vi "JSONtext Multi-step Filter.vi"() -> ()   [LabVIEW 2017] (continued)
laborum. Quis sint fugiat deserunt incididunt enim sit magna occaecat mollit.\\r\\n\",\n    \"registered\": \"2014-01-11T05:01:09 -00:00\",\n    \"latitude\": -55.686363,\n    \"longitude\": -121.895445,\n    \"tags\": [\n      \"nostrud\",\n      \"adipisicing\",\n      \"proident\",\n      \"reprehenderit\",\n      \"minim\",\n      \"incididunt\",\n      \"do\"\n    ],\n    \"friends\": [\n      {\n        \"id\": 0,\n        \"name\": \"Bowman Haynes\"\n      },\n      {\n        \"id\": 1,\n        \"name\": \"Rosalind Dejesus\"\n      },\n      {\n        \"id\": 2,\n        \"name\": \"Mayra Finch\"\n      }\n    ],\n    \"greeting\": \"Hello, Agnes Frye! You have 4 unread messages.\",\n    \"favoriteFruit\": \"apple\"\n  },\n  {\n    \"_id\": \"59b53bcb9737cc098f392507\",\n    \"index\": 79,\n    \"guid\": \"14e019ee-c0ef-4d9f-a34b-1e266fe4f201\",\n    \"isActive\": true,\n    \"balance\": \"$2,153.21\",\n    \"picture\": \"http://placehold.it/32x32\",\n    \"age\": 36,\n    \"eyeColor\": \"blue\",\n    \"name\": \"Edwards Dennis\",\n    \"gender\": \"male\",\n    \"company\": \"ARCTIQ\",\n    \"email\": \"edwardsdennis@arctiq.com\",\n    \"phone\": \"+1 (883) 475-3655\",\n    \"address\": \"269 Melba Court, Soudan, Oregon, 9327\",\n    \"about\": \"Fugiat exercitation sit est excepteur enim culpa. Adipisicing fugiat labore adipisicing fugiat commodo minim. Dolor amet nisi ea deserunt nisi consequat. Duis aliqua in qui veniam exercitation officia labore amet fugiat. Dolore deserunt ullamco quis esse enim incididunt cupidatat. Dolore in laborum dolor id in mollit esse ut sit laborum deserunt duis consequat. Aliqua consectetur nulla esse ad laborum est amet veniam incididunt est anim cillum ad reprehenderit.\\r\\n\",\n    \"registered\": \"2014-11-20T11:02:11 -00:00\",\n    \"latitude\": 4.916048,\n    \"longitude\": 67.818849,\n    \"tags\": [\n      \"ipsum\",\n      \"ea\",\n      \"nisi\",\n      \"fugiat\",\n      \"qui\",\n      \"occaecat\",\n      \"duis\"\n    ],\n    \"friends\": [\n      {\n        \"id\": 0,\n        \"name\": \"Pearson Obrien\"\n      },\n      {\n        \"id\": 1,\n        \"name\": \"Jaime Castillo\"\n      },\n      {\n        \"id\": 2,\n        \"name\": \"Fowler Branch\"\n      }\n    ],\n    \"greeting\": \"Hello, Edwards Dennis! You have 3 unread messages.\",\n    \"favoriteFruit\": \"apple\"\n  },\n  {\n    \"_id\": \"59b53bcbc88425d302bb5dc9\",\n    \"index\": 80,\n    \"guid\": \"8d66411d-3632-46fa-adba-de988295c355\",\n    \"isActive\": true,\n    \"balance\": \"$1,048.45\",\n    \"picture\": \"http://placehold.it/32x32\",\n    \"age\": 20,\n    \"eyeColor\": \"brown\",\n    \"name\": \"Tonya Harrell\",\n    \"gender\": \"female\",\n    \"company\": \"MIRACLIS\",\n    \"email\": \"tonyaharrell@miraclis.com\",\n    \"phone\": \"+1 (955) 521-2821\",\n    \"address\": \"458 Hart Street, Otranto, Florida, 9320\",\n    \"about\": \"Sit laboris tempor do reprehenderit. Reprehenderit exercitation consectetur aliquip nisi nisi occaecat magna magna pariatur. Reprehenderit eiusmod cillum irure aliqua laboris dolore occaecat anim commodo ad dolore. Laborum fugiat minim pariatur sunt enim qui cupidatat labore ex esse cupidatat id aliquip.\\r\\n\",\n    \"registered\": \"2016-08-02T02:36:17 -01:00\",\n    \"latitude\": 60.952856,\n    \"longitude\": 45.278246,\n    \"tags\": [\n      \"minim\",\n      \"nulla\",\n      \"laboris\",\n      \"exercitation\",\n      \"duis\",\n      \"eiusmod\",\n      \"amet\"\n    ],\n    \"friends\": [\n      {\n        \"id\": 0,\n        \"name\": \"Clara Harding\"\n      },\n      {\n        \"id\": 1,\n        \"name\": \"Corine Lindsey\"\n      },\n      {\n        \"id\": 2,\n        \"name\": \"Mcfarland Martinez\"\n      }\n    ],\n    \"greeting\": \"Hello, Tonya Harrell! You have 2 unread messages.\",\n    \"favoriteFruit\": \"strawberry\"\n  },\n  {\n    \"_id\": \"59b53bcb6dc7404c96b23788\",\n    \"index\": 81,\n    \"guid\": \"d16339bd-0d5a-4fda-9a80-3523f38c2607\",\n    \"isActive\": false,\n    \"balance\": \"$3,172.05\",\n    \"picture\": \"http://placehold.it/32x32\",\n    \"age\": 26,\n    \"eyeColor\": \"blue\",\n    \"name\": \"Robertson Malone\",\n    \"gender\": \"male\",\n    \"company\": \"UNIA\",\n    \"email\": \"robertsonmalone@unia.com\",\n    \"phone\": \"+1 (962) 481-2396\",\n    \"address\": \"590 Newel Street, Joppa, Minnesota, 5936\",\n    \"about\": \"Do duis laboris elit dolor amet exercitation. Irure aliqua veniam consectetur culpa enim in officia voluptate ad. Adipisicing sint do et commodo. Culpa in adipisicing voluptate aliqua Lorem exercitation sunt ullamco pariatur voluptate mollit aliquip. Laboris quis labore minim officia. Dolor Lorem tempor aute minim commodo duis incididunt laboris enim sit sint mollit.\\r\\n\",\n    \"registered\": \"2016-07-26T05:07:36 -01:00\",\n    \"latitude\": 74.88141,\n    \"longitude\": -149.072395,\n    \"tags\": [\n      \"sit\",\n      \"commodo\",\n      \"Lorem\",\n      \"ex\",\n      \"fugiat\",\n      \"fugiat\",\n      \"dolor\"\n    ],\n    \"friends\": [\n      {\n        \"id\": 0,\n        \"name\": \"Winifred Tate\"\n      },\n      {\n        \"id\": 1,\n        \"name\": \"Curtis Reid\"\n      },\n      {\n        \"id\": 2,\n        \"name\": \"Chase Keith\"\n      }\n    ],\n    \"greeting\": \"Hello, Robertson Malone! You have 7 unread messages.\",\n    \"favoriteFruit\": \"apple\"\n  },\n  {\n    \"_id\": \"59b53bcb51c65aa434aa3d1f\",\n    \"index\": 82,\n    \"guid\": \"2774080d-3b85-4a4f-97f3-157e9148c011\",\n    \"isActive\": true,\n    \"balance\": \"$3,693.94\",\n    \"picture\": \"http://placehold.it/32x32\",\n    \"age\": 21,\n    \"eyeColor\": \"blue\",\n    \"name\": \"Mercedes Leonard\",\n    \"gender\": \"female\",\n    \"company\": \"MIRACULA\",\n    \"email\": \"mercedesleonard@miracula.com\",\n    \"phone\": \"+1 (847) 435-3340\",\n    \"address\": \"900 Grafton Street, Mulberry, Hawaii, 4401\",\n    \"about\": \"Consectetur laborum eu occaecat occaecat id minim. Duis do veniam adipisicing voluptate consectetur labore quis elit. Cillum dolore ex fugiat deserunt sint ea magna cillum reprehenderit amet consectetur proident. Culpa ut cillum nulla sit voluptate voluptate veniam qui. Ut anim minim pariatur velit dolor cupidatat ut. Irure Lorem fugiat incididunt ad cillum sit nisi sunt sint dolor elit. Elit non minim laborum ex dolor commodo labore quis irure officia duis labore.\\r\\n\",\n    \"registered\": \"2015-09-07T03:13:08 -01:00\",\n    \"latitude\": -37.746734,\n    \"longitude\": 158.145458,\n    \"tags\": [\n      \"ipsum\",\n      \"dolor\",\n      \"occaecat\",\n      \"aute\",\n      \"dolor\",\n      \"ex\",\n      \"id\"\n    ],\n    \"friends\": [\n      {\n        \"id\": 0,\n        \"name\": \"Jerri Miller\"\n      },\n      {\n        \"id\": 1,\n        \"name\": \"Huff Pitts\"\n      },\n      {\n        \"id\": 2,\n        \"name\": \"Kristine Pittman\"\n      }\n    ],\n    \"greeting\": \"Hello, Mercedes Leonard! You have 7 unread messages.\",\n    \"favoriteFruit\": \"apple\"\n  },\n  {\n    \"_id\": \"59b53bcbb5cb7bde1ba115a7\",\n    \"index\": 83,\n    \"guid\": \"5fa9bb18-fd83-47f9-8f54-1c8eab99fa1f\",\n    \"isActive\": false,\n    \"balance\": \"$2,449.67\",\n    \"picture\": \"http://placehold.it/32x32\",\n    \"age\": 27,\n    \"eyeColor\": \"brown\",\n    \"name\": \"Rebekah Cardenas\",\n    \"gender\": \"female\",\n    \"company\": \"MEDCOM\",\n    \"email\": \"rebekahcardenas@medcom.com\",\n    \"phone\": \"+1 (930) 526-2666\",\n    \"address\": \"585 Conduit Boulevard, Edenburg, Pennsylvania, 5520\",\n    \"about\": \"Sint magna ad consequat cupidatat ut quis duis ut deserunt duis sit consequat. Nisi ea ad ex occaecat adipisicing voluptate quis aliquip nostrud amet quis. Veniam consectetur amet magna adipisicing commodo ea esse elit occaecat labore pariatur. Adipisicing laboris Lorem sit incididunt pariatur eu. Do ipsum laborum excepteur cillum in.\\r\\n\",\n    \"registered\": \"2015-04-23T12:08:15 -01:00\",\n    \"latitude\": -70.810485,\n    \"longitude\": -5.673714,\n    \"tags\": [\n      \"eu\",\n      \"elit\",\n      \"do\",\n      \"laboris\",\n      \"eu\",\n      \"pariatur\",\n      \"sunt\"\n    ],\n    \"friends\": [\n      {\n        \"id\": 0,\n        \"name\": \"Selma Hughes\"\n      },\n      {\n        \"id\": 1,\n        \"name\": \"Laverne Ware\"\n      },\n      {\n        \"id\": 2,\n        \"name\": \"Cortez Reilly\"\n      }\n    ],\n    \"greeting\": \"Hello, Rebekah Cardenas! You have 5 unread messages.\",\n    \"favoriteFruit\": \"strawberry\"\n  },\n  {\n    \"_id\": \"59b53bcbf398f609774512fb\",\n    \"index\": 84,\n    \"guid\": \"9798106c-d85b-4df5-a840-9220e34cb34d\",\n    \"isActive\": true,\n    \"balance\": \"$3,845.69\",\n    \"picture\": \"http://placehold.it/32x32\",\n    \"age\": 28,\n    \"eyeColor\": \"brown\",\n    \"name\": \"Rena Norman\",\n    \"gender\": \"female\",\n    \"company\": \"AQUOAVO\",\n    \"email\": \"renanorman@aquoavo.com\",\n    \"phone\": \"+1 (983) 520-2908\",\n    \"address\": \"635 Cedar Street, Richford, Virginia, 7412\",\n    \"about\": \"Id incididunt in veniam officia nisi veniam dolore laboris duis. Eu dolore labore excepteur tempor exercitation pariatur est commodo elit ullamco quis voluptate. Culpa magna anim ad nisi cupidatat proident dolor sit esse aute reprehenderit deserunt id non. Aliquip consequat nulla aliqua mollit dolore nostrud officia amet pariatur commodo proident. Dolore occaecat ex cupidatat ea exercitation velit amet. Laborum officia non anim ea eiusmod tempor consequat laboris est enim culpa irure enim. Sit dolor dolore dolore nisi magna deserunt sint culpa est excepteur aute.\\r\\n\",\n    \"registered\": \"2015-12-14T03:36:58 -00:00\",\n    \"latitude\": -35.296091,\n    \"longitude\": 130.813918,\n    \"tags\": [\n      \"laboris\",\n      \"nisi\",\n      \"ipsum\",\n      \"qui\",\n      \"reprehenderit\",\n      \"ipsum\",\n      \"incididunt\"\n    ],\n    \"friends\": [\n      {\n        \"id\": 0,\n        \"name\": \"Fry Pace\"\n      },\n      {\n        \"id\": 1,\n        \"name\": \"Levy Norton\"\n      },\n      {\n        \"id\": 2,\n        \"name\": \"Lupe Snider\"\n      }\n    ],\n    \"greeting\": \"Hello, Rena Norman! You have 3 unread messages.\",\n    \"favoriteFruit\": \"banana\"\n  },\n  {\n    \"_id\": \"59b53bcb388b74959570b328\",\n    \"index\": 85,\n    \"guid\": \"ef150b45-285d-447c-8120-8e1ae6b7ddb0\",\n    \"isActive\": false,\n    \"balance\": \"$3,528.91\",\n    \"picture\": \"http://placehold.it/32x32\",\n    \"age\": 33,\n    \"eyeColor\": \"green\",\n    \"name\": \"Russell Hunter\",\n    \"gender\": \"male\",\n    \"company\": \"KONNECT\",\n    \"email\": \"russellhunter@konnect.com\",\n    \"phone\": \"+1 (923) 579-2669\",\n    \"address\": \"991 Agate Court, Westwood, Kansas, 7904\",\n    \"about\": \"Mollit officia duis anim laborum et sunt dolor commodo est fugiat. Cillum ipsum minim irure ea pariatur officia non deserunt aliqua sit Lorem veniam. Cillum amet deserunt occaecat eiusmod magna esse mollit. Eiusmod fugiat et cillum minim ullamco velit sint enim qui exercitation. Magna nostrud deserunt adipisicing nisi ullamco quis culpa aliquip voluptate do.\\r\\n\",\n    \"registered\": \"2014-01-24T12:47:30 -00:00\",\n    \"latitude\": -4.402596,\n    \"longitude\": -44.068437,\n    \"tags\": [\n      \"duis\",\n      \"aliqua\",\n      \"aliquip\",\n      \"ullamco\",\n      \"nulla\",\n      \"anim\",\n      \"eiusmod\"\n    ],\n    \"friends\": [\n      {\n        \"id\": 0,\n        \"name\": \"Jolene Bonner\"\n      },\n      {\n        \"id\": 1,\n        \"name\": \"Head Calhoun\"\n      },\n      {\n        \"id\": 2,\n        \"name\": \"Kate Reyes\"\n      }\n    ],\n    \"greeting\": \"Hello, Russell Hunter! You have 6 unread messages.\",\n    \"favoriteFruit\": \"strawberry\"\n  },\n  {\n    \"_id\": \"59b53bcb2db0467411e874a7\",\n    \"index\": 86,\n    \"guid\": \"c8749167-fdd7-4919-911e-bf0b7c47fa22\",\n    \"isActive\": true,\n    \"balance\": \"$3,021.98\",\n    \"picture\": \"http://placehold.it/32x32\",\n    \"age\": 30,\n    \"eyeColor\": \"green\",\n    \"name\": \"Singleton May\",\n    \"gender\": \"male\",\n    \"company\": \"OBONES\",\n    \"email\": \"singletonmay@obones.com\",\n    \"phone\": \"+1 (809) 470-2340\",\n    \"address\": \"513 Stuyvesant Avenue, Fairlee, Puerto Rico, 6772\",\n    \"about\": \"Ea irure Lorem nulla duis do do et nostrud exercitation. Voluptate exercitation aute consequat eu est. Et cillum labore consectetur amet. Ea pariatur magna et excepteur anim sit pariatur occaecat velit sunt veniam anim.\\r\\n\",\n    \"registered\": \"2016-04-15T10:43:19 -01:00\",\n    \"latitude\": -67.961908,\n    \"longitude\": -28.926166,\n    \"tags\": [\n      \"consequat\",\n      \"pariatur\",\n      \"tempor\",\n      \"et\",\n      \"excepteur\",\n      \"incididunt\",\n      \"tempor\"\n    ],\n    \"friends\": [\n      {\n        \"id\": 0,\n        \"name\": \"Mendoza Estes\"\n      },\n      {\n        \"id\": 1,\n        \"name\": \"Bean Bolton\"\n      },\n      {\n        \"id\": 2,\n        \"name\": \"Holder Villarreal\"\n      }\n    ],\n    \"greeting\": \"Hello, Singleton May! You have 3 unread messages.\",\n    \"favoriteFruit\": \"apple\"\n  },\n  {\n    \"_id\": \"59b53bcbaefe5ada14509d19\",\n    \"index\": 87,\n    \"guid\": \"ead04019-6a40-4420-a798-b8883cd03185\",\n    \"isActive\": true,\n    \"balance\": \"$1,396.19\",\n    \"picture\": \"http://placehold.it/32x32\",\n    \"age\": 39,\n    \"eyeColor\": \"blue\",\n    \"name\": \"Jewell Bradshaw\",\n    \"gender\": \"female\",\n    \"company\": \"JUMPSTACK\",\n    \"email\": \"jewellbradshaw@jumpstack.com\",\n    \"phone\": \"+1 (968) 458-2531\",\n    \"address\": \"782 Winthrop Street, Dotsero, South Carolina, 5062\",\n    \"about\": \"Amet deserunt pariatur in elit exercitation labore. Quis dolore Lorem pariatur irure tempor amet culpa duis enim deserunt exercitation proident. Nostrud magna qui irure dolore est excepteur magna nulla ipsum anim ullamco. Velit occaecat sunt exercitation minim consequat. Eu sunt cillum non amet pariatur mollit sunt amet ad non irure.\\r\\n\",\n    \"registered\": \"2014-09-14T04:22:20 -01:00\",\n    \"latitude\": 29.814291,\n    \"longitude\": 61.37831,\n    \"tags\": [\n      \"sint\",\n      \"elit\",\n      \"ad\",\n      \"ad\",\n      \"cupidatat\",\n      \"cillum\",\n      \"sit\"\n    ],\n    \"friends\": [\n      {\n        \"id\": 0,\n        \"name\": \"Rosales Richmond\"\n      },\n      {\n        \"id\": 1,\n        \"name\": \"Sara Duffy\"\n      },\n      {\n        \"id\": 2,\n        \"name\": \"Freida Pollard\"\n      }\n    ],\n    \"greeting\": \"Hello, Jewell Bradshaw! You have 10 unread messages.\",\n    \"favoriteFruit\": \"strawberry\"\n  },\n  {\n    \"_id\": \"59b53bcb431347b2e14132f2\",\n    \"index\": 88,\n    \"guid\": \"caf8be88-33b4-4c13-8fba-e0e573a30583\",\n    \"isActive\": true,\n    \"balance\": \"$1,502.06\",\n    \"picture\": \"http://placehold.it/32x32\",\n    \"age\": 40,\n    \"eyeColor\": \"blue\",\n    \"name\": \"Langley Bauer\",\n    \"gender\": \"male\",\n    \"company\": \"PORTICA\",\n    \"email\": \"langleybauer@portica.com\",\n    \"phone\": \"+1 (980) 600-2629\",\n    \"address\": \"193 George Street, Navarre, Mississippi, 3789\",\n    \"about\": \"Exercitation irure ad magna sunt consequat non. Do amet tempor consequat adipisicing reprehenderit sunt. Do ipsum aliquip dolore amet ullamco. Eu proident reprehenderit consequat velit. Exercitation minim eiusmod quis incididunt magna magna exercitation consectetur irure.\\r\\n\",\n    \"registered\": \"2015-12-09T03:10:32 -00:00\",\n    \"latitude\": 14.711439,\n    \"longitude\": 101.330203,\n    \"tags\": [\n      \"sunt\",\n      \"laboris\",\n      \"nisi\",\n      \"velit\",\n      \"ipsum\",\n      \"fugiat\",\n      \"amet\"\n    ],\n    \"friends\": [\n      {\n        \"id\": 0,\n        \"name\": \"Noble Odom\"\n      },\n      {\n        \"id\": 1,\n        \"name\": \"Mara Everett\"\n      },\n      {\n        \"id\": 2,\n        \"name\": \"Carole Benson\"\n      }\n    ],\n    \"greeting\": \"Hello, Langley Bauer! You have 1 unread messages.\",\n    \"favoriteFruit\": \"apple\"\n  },\n  {\n    \"_id\": \"59b53bcb9cfbbb3d3b86db36\",\n    \"index\": 89,\n    \"guid\": \"585ace61-13af-493d-9fa6-61d9246efb80\",\n    \"isActive\": true,\n    \"balance\": \"$2,788.64\",\n    \"picture\": \"http://placehold.it/32x32\",\n    \"age\": 39,\n    \"eyeColor\": \"green\",\n    \"name\": \"Walker Sandoval\",\n    \"gender\": \"male\",\n    \"company\": \"EXPOSA\",\n    \"email\": \"walkersandoval@exposa.com\",\n    \"phone\": \"+1 (813) 589-3863\",\n    \"address\": \"597 Dunham Place, Albrightsville, Wisconsin, 6040\",\n    \"about\": \"Cillum ipsum velit ea esse cupidatat aliquip deserunt. Velit labore enim et et dolor esse duis voluptate Lorem ea. Esse Lorem excepteur quis cillum mollit anim voluptate fugiat est culpa. Ullamco Lorem fugiat tempor sunt incididunt aliquip occaecat mollit sit aliqua velit. Ex ullamco consequat minim minim do sint commodo anim fugiat do. Cupidatat id nulla in adipisicing magna consequat deserunt cillum. Ad id occaecat mollit id ullamco.\\r\\n\",\n    \"registered\": \"2016-04-14T12:25:38 -01:00\",\n    \"latitude\": -16.535757,\n    \"longitude\": -28.076556,\n    \"tags\": [\n      \"consectetur\",\n      \"commodo\",\n      \"magna\",\n      \"duis\",\n      \"cillum\",\n      \"id\",\n      \"mollit\"\n    ],\n    \"friends\": [\n      {\n        \"id\": 0,\n        \"name\": \"Tamra Watson\"\n      },\n      {\n        \"id\": 1,\n        \"name\": \"Deidre Gamble\"\n      },\n      {\n        \"id\": 2,\n        \"name\": \"Graham Harris\"\n      }\n    ],\n    \"greeting\": \"Hello, Walker Sandoval! You have 6 unread messages.\",\n    \"favoriteFruit\": \"banana\"\n  },\n  {\n    \"_id\": \"59b53bcb4f8125393e1be565\",\n    \"index\": 90,\n    \"guid\": \"50b5a169-63ec-430b-bd65-956e383c7b25\",\n    \"isActive\": true,\n    \"balance\": \"$2,863.84\",\n    \"picture\": \"http://placehold.it/32x32\",\n    \"age\": 33,\n    \"eyeColor\": \"brown\",\n    \"name\": \"Carlene Humphrey\",\n    \"gender\": \"female\",\n    \"company\": \"WEBIOTIC\",\n    \"email\": \"carlenehumphrey@webiotic.com\",\n    \"phone\": \"+1 (957) 535-2883\",\n    \"address\": \"367 Kensington Street, Carrizo, Indiana, 3136\",\n    \"about\": \"Voluptate pariatur ex pariatur duis non quis ex cillum. Labore occaecat tempor in enim proident aliquip. Consequat ex veniam ullamco aute aute cupidatat dolor dolore ad velit incididunt.\\r\\n\",\n    \"registered\": \"2015-09-17T11:41:14 -01:00\",\n    \"latitude\": -25.860369,\n    \"longitude\": 159.878255,\n    \"tags\": [\n      \"eiusmod\",\n      \"consectetur\",\n      \"consectetur\",\n      \"id\",\n      \"id\",\n      \"eiusmod\",\n      \"ad\"\n    ],\n    \"friends\": [\n      {\n        \"id\": 0,\n        \"name\": \"Baird Reed\"\n      },\n      {\n        \"id\": 1,\n        \"name\": \"Dollie Stephens\"\n      },\n      {\n        \"id\": 2,\n        \"name\": \"Greta Buckley\"\n      }\n    ],\n    \"greeting\": \"Hello, Carlene Humphrey! You have 6 unread messages.\",\n    \"favoriteFruit\": \"banana\"\n  },\n  {\n    \"_id\": \"59b53bcb68c2646e78378cd5\",\n    \"index\": 91,\n    \"guid\": \"ea0a37f9-d18f-4eba-8810-ab098ee81cd3\",\n    \"isActive\": true,\n    \"balance\": \"$1,333.07\",\n    \"picture\": \"http://placehold.it/32x32\",\n    \"age\": 22,\n    \"eyeColor\": \"brown\",\n    \"name\": \"Mattie Mckinney\",\n    \"gender\": \"female\",\n    \"company\": \"PATHWAYS\",\n    \"email\": \"mattiemckinney@pathways.com\",\n    \"phone\": \"+1 (985) 530-3103\",\n    \"address\": \"803 Taaffe Place, Brutus, Tennessee, 1065\",\n    \"about\": \"Aute aute ipsum nostrud commodo. Elit laboris magna irure id laboris eu et nisi. Sit ipsum irure deserunt voluptate nisi ut ut. Aute ullamco deserunt ex elit in et qui excepteur aliquip. Dolore id veniam irure irure anim irure ex exercitation id ea.\\r\\n\",\n    \"registered\": \"2014-11-08T08:00:06 -00:00\",\n    \"latitude\": -3.533773,\n    \"longitude\": -136.23028,\n    \"tags\": [\n      \"sit\",\n      \"excepteur\",\n      \"esse\",\n      \"fugiat\",\n      \"proident\",\n      \"id\",\n      \"veniam\"\n    ],\n    \"friends\": [\n      {\n        \"id\": 0,\n        \"name\": \"Latonya Wright\"\n      },\n      {\n        \"id\": 1,\n        \"name\": \"Mable Estrada\"\n      },\n      {\n        \"id\": 2,\n        \"name\": \"Estelle Henson\"\n      }\n    ],\n    \"greeting\": \"Hello, Mattie Mckinney! You have 2 unread messages.\",\n    \"favoriteFruit\": \"strawberry\"\n  },\n  {\n    \"_id\": \"59b53bcb88186672d782d77f\",\n    \"index\": 92,\n    \"guid\": \"63483e35-f63f-47ea-904f-a48dcde71fb1\",\n    \"isActive\": false,\n    \"balance\": \"$3,958.35\",\n    \"picture\": \"http://placehold.it/32x32\",\n    \"age\": 22,\n    \"eyeColor\": \"green\",\n    \"name\": \"Tamara Russo\",\n    \"gender\": \"female\",\n    \"company\": \"EBIDCO\",\n    \"email\": \"tamararusso@ebidco.com\",\n    \"phone\": \"+1 (941) 482-2355\",\n    \"address\": \"184 Dumont Avenue, Chumuckla, Georgia, 7344\",\n    \"about\": \"Tempor cupidatat labore excepteur irure velit sunt aliqua aliquip ea qui. Deserunt mollit cupidatat non amet exercitation eu proident. Occaecat excepteur aliqua exercitation irure dolor. Eiusmod adipisicing incididunt reprehenderit anim proident nulla cupidatat anim. In non consectetur laborum adipisicing nostrud. Eiusmod mollit voluptate aute et ut est voluptate enim laborum occaecat incididunt.\\r\\n\",\n    \"registered\": \"2014-01-11T06:03:38 -00:00\",\n    \"latitude\": 4.570218,\n    \"longitude\": 97.967557,\n    \"tags\": [\n      \"adipisicing\",\n      \"occaecat\",\n      \"tempor\",\n      \"anim\",\n      \"commodo\",\n      \"do\",\n      \"ea\"\n    ],\n    \"friends\": [\n      {\n        \"id\": 0,\n        \"name\": \"Suzette Burch\"\n      },\n      {\n        \"id\": 1,\n        \"name\": \"Velazquez Mayer\"\n      },\n      {\n        \"id\": 2,\n        \"name\": \"Shannon Powell\"\n      }\n    ],\n    \"greeting\": \"Hello, Tamara Russo! You have 9 unread messages.\",\n    \"favoriteFruit\": \"banana\"\n  },\n  {\n    \"_id\": \"59b53bcb9c166135e4f617f9\",\n    \"index\": 93,\n    \"guid\": \"93bacd52-b79c-429e-8685-45799e149002\",\n    \"isActive\": false,\n    \"balance\": \"$2,892.53\",\n    \"picture\": \"http://placehold.it/32x32\",\n    \"age\": 22,\n    \"eyeColor\": \"brown\",\n    \"name\": \"Camacho Talley\",\n    \"gender\": \"male\",\n    \"company\": \"GRAINSPOT\",\n    \"email\": \"camachotalley@grainspot.com\",\n    \"phone\": \"+1 (877) 502-3157\",\n    \"address\": \"977 Roosevelt Court, Gila, New Hampshire, 5370\",\n    \"about\": \"Duis nulla culpa cupidatat amet amet qui. Ut sit dolor laboris quis ullamco. Aute nulla aliqua voluptate fugiat labore ut. Sunt veniam veniam duis commodo pariatur. Commodo occaecat anim ad est aliquip.\\r\\n\",\n    \"registered\": \"2014-09-29T05:59:11 -01:00\",\n    \"latitude\": 65.471967,\n    \"longitude\": -142.24607,\n    \"tags\": [\n      \"id\",\n      \"aute\",\n      \"magna\",\n      \"eiusmod\",\n      \"mollit\",\n      \"ipsum\",\n      \"commodo\"\n    ],\n    \"friends\": [\n      {\n        \"id\": 0,\n        \"name\": \"Hopkins Atkins\"\n      },\n      {\n        \"id\": 1,\n        \"name\": \"Mcclain Santos\"\n      },\n      {\n        \"id\": 2,\n        \"name\": \"Enid Kemp\"\n      }\n    ],\n    \"greeting\": \"Hello, Camacho Talley! You have 5 unread messages.\",\n    \"favoriteFruit\": \"strawberry\"\n  },\n  {\n    \"_id\": \"59b53bcbe2a5bd209ec5b3c8\",\n    \"index\": 94,\n    \"guid\": \"036605db-b6ec-42e9-a1bc-ee2f3b70a5df\",\n    \"isActive\": false,\n    \"balance\": \"$3,938.69\",\n    \"picture\": \"http://placehold.it/32x32\",\n    \"age\": 38,\n    \"eyeColor\": \"green\",\n    \"name\": \"Barbra Morton\",\n    \"gender\": \"female\",\n    \"company\": \"DANJA\",\n    \"email\": \"barbramorton@danja.com\",\n    \"phone\": \"+1 (948) 444-3914\",\n    \"address\": \"970 Rutherford Place, Selma, Louisiana, 3091\",\n    \"about\": \"Proident labore esse non enim consequat laboris quis irure pariatur enim. Aliquip veniam id occaecat laborum consectetur proident ea cillum amet consequat in id. Esse fugiat veniam ullamco culpa exercitation. Pariatur deserunt consectetur qui consectetur aliquip ea irure eiusmod. Ipsum sint ad ex id. Veniam laborum quis cillum qui quis exercitation qui aliquip mollit eiusmod.\\r\\n\",\n    \"registered\": \"2017-08-11T12:43:09 -01:00\",\n    \"latitude\": 36.516788,\n    \"longitude\": 150.180024,\n    \"tags\": [\n      \"tempor\",\n      \"id\",\n      \"aliquip\",\n      \"sit\",\n      \"dolore\",\n      \"qui\",\n      \"nulla\"\n    ],\n    \"friends\": [\n      {\n        \"id\": 0,\n        \"name\": \"Benton Boyle\"\n      },\n      {\n        \"id\": 1,\n        \"name\": \"Bates Mejia\"\n      },\n      {\n        \"id\": 2,\n        \"name\": \"Montoya Weber\"\n      }\n    ],\n    \"greeting\": \"Hello, Barbra Morton! You have 3 unread messages.\",\n    \"favoriteFruit\": \"strawberry\"\n  },\n  {\n    \"_id\": \"59b53bcb7e036dc098f119d8\",\n    \"index\": 95,\n    \"guid\": \"acd5167b-c778-494e-9b08-c3867c5930d5\",\n    \"isActive\": true,\n    \"balance\": \"$3,887.96\",\n    \"picture\": \"http://placehold.it/32x32\",\n    \"age\": 28,\n    \"eyeColor\": \"blue\",\n    \"name\": \"Andrea Barton\",\n    \"gender\": \"female\",\n    \"company\": \"TRIPSCH\",\n    \"email\": \"andreabarton@tripsch.com\",\n    \"phone\": \"+1 (839) 508-3740\",\n    \"address\": \"531 Elm Place, Choctaw, Oklahoma, 4348\",\n    \"about\": \"Aute ullamco laborum esse quis voluptate enim amet consectetur non incididunt nostrud anim sit ea. Quis eiusmod reprehenderit tempor ea aliquip. Magna laboris pariatur id aliqua nostrud labore incididunt ut.\\r\\n\",\n    \"registered\": \"2017-01-18T09:09:30 -00:00\",\n    \"latitude\": 87.073078,\n    \"longitude\": -153.089878,\n    \"tags\": [\n      \"minim\",\n      \"deserunt\",\n      \"proident\",\n      \"dolore\",\n      \"sunt\",\n      \"excepteur\",\n      \"ea\"\n    ],\n    \"friends\": [\n      {\n        \"id\": 0,\n        \"name\": \"Samantha Carrillo\"\n      },\n      {\n        \"id\": 1,\n        \"name\": \"Burke Mckenzie\"\n      },\n      {\n        \"id\": 2,\n        \"name\": \"Alford Love\"\n      }\n    ],\n    \"greeting\": \"Hello, Andrea Barton! You have 6 unread messages.\",\n    \"favoriteFruit\": \"strawberry\"\n  },\n  {\n    \"_id\": \"59b53bcbe68489b710be92d8\",\n    \"index\": 96,\n    \"guid\": \"fcdbceb5-35bc-464d-9cda-0730a96ae61d\",\n    \"isActive\": false,\n    \"balance\": \"$3,067.07\",\n    \"picture\": \"http://placehold.it/32x32\",\n    \"age\": 29,\n    \"eyeColor\": \"blue\",\n    \"name\": \"Edna Simpson\",\n    \"gender\": \"female\",\n    \"company\": \"TYPHONICA\",\n    \"email\": \"ednasimpson@typhonica.com\",\n    \"phone\": \"+1 (887) 582-2829\",\n    \"address\": \"169 Dictum Court, Callaghan, Alaska, 6930\",\n    \"about\": \"Elit veniam ea culpa do nulla consequat culpa ad sunt enim. Laborum aliqua voluptate incididunt magna aliqua consectetur officia consequat anim fugiat aliquip proident cillum. Sunt proident occaecat dolore aute tempor labore minim consectetur. Esse mollit velit id aute minim eiusmod labore cillum. Adipisicing aliquip minim cupidatat nulla aliquip eiusmod quis ut nulla occaecat nulla cupidatat. Tempor laboris consectetur reprehenderit mollit eu cillum pariatur laboris commodo enim Lorem officia.\\r\\n\",\n    \"registered\": \"2016-05-10T05:37:46 -01:00\",\n    \"latitude\": -30.023422,\n    \"longitude\": 0.886087,\n    \"tags\": [\n      \"in\",\n      \"id\",\n      \"officia\",\n      \"anim\",\n      \"labore\",\n      \"ad\",\n      \"sunt\"\n    ],\n    \"friends\": [\n      {\n        \"id\": 0,\n        \"name\": \"Lina Brown\"\n      },\n      {\n        \"id\": 1,\n        \"name\": \"Cain Campos\"\n      },\n      {\n        \"id\": 2,\n        \"name\": \"Sparks Jones\"\n      }\n    ],\n    \"greeting\": \"Hello, Edna Simpson! You have 10 unread messages.\",\n    \"favoriteFruit\": \"banana\"\n  },\n  {\n    \"_id\": \"59b53bcbcfbbc8d0511541f4\",\n    \"index\": 97,\n    \"guid\": \"7281cfd2-d40d-48e4-957e-b86b371683a2\",\n    \"isActive\": true,\n    \"balance\": \"$2,179.76\",\n    \"picture\": \"http://placehold.it/32x32\",\n    \"age\": 35,\n    \"eyeColor\": \"brown\",\n    \"name\": \"Charlene Woods\",\n    \"gender\": \"female\",\n    \"company\": \"JUNIPOOR\",\n    \"email\": \"charlenewoods@junipoor.com\",\n    \"phone\": \"+1 (919) 557-3560\",\n    \"address\": \"161 Tabor Court, Itmann, North Dakota, 9686\",\n    \"about\": \"Mollit velit cillum irure Lorem id consectetur fugiat. Reprehenderit ipsum aliquip tempor dolor. Eu reprehenderit tempor adipisicing anim duis non quis officia excepteur fugiat sunt adipisicing. Consectetur qui aliquip eiusmod laborum do incididunt id ipsum sint est elit ad commodo. Adipisicing veniam eu tempor id et nisi fugiat. Qui duis aute fugiat qui ut id ut deserunt adipisicing aliqua. Fugiat aliqua incididunt Lorem esse ipsum elit magna quis eiusmod pariatur.\\r\\n\",\n    \"registered\": \"2014-09-19T12:55:15 -01:00\",\n    \"latitude\": 23.852484,\n    \"longitude\": 64.974725,\n    \"tags\": [\n      \"deserunt\",\n      \"pariatur\",\n      \"nulla\",\n      \"qui\",\n      \"nulla\",\n      \"proident\",\n      \"aliquip\"\n    ],\n    \"friends\": [\n      {\n        \"id\": 0,\n        \"name\": \"Rachael Cabrera\"\n      },\n      {\n        \"id\": 1,\n        \"name\": \"Best Huber\"\n      },\n      {\n        \"id\": 2,\n        \"name\": \"Luann Abbott\"\n      }\n    ],\n    \"greeting\": \"Hello, Charlene Woods! You have 2 unread messages.\",\n    \"favoriteFruit\": \"banana\"\n  },\n  {\n    \"_id\": \"59b53bcb678a7787e8012db4\",\n    \"index\": 98,\n    \"guid\": \"7519df16-5d86-4a4e-a0b6-19e2f100d49d\",\n    \"isActive\": true,\n    \"balance\": \"$3,153.52\",\n    \"picture\": \"http://placehold.it/32x32\",\n    \"age\": 31,\n    \"eyeColor\": \"blue\",\n    \"name\": \"Pugh Christensen\",\n    \"gender\": \"male\",\n    \"company\": \"PLEXIA\",\n    \"email\": \"pughchristensen@plexia.com\",\n    \"phone\": \"+1 (803) 541-2906\",\n    \"address\": \"514 Wyckoff Avenue, Concho, Washington, 1004\",\n    \"about\": \"Fugiat duis nisi esse duis ut tempor laborum amet. Ut et labore quis pariatur ullamco deserunt esse occaecat est pariatur. Ut cillum pariatur nulla dolor eu consequat nisi nisi occaecat occaecat ad veniam commodo. Cillum anim eu fugiat minim excepteur dolor sit. Dolore aute ipsum qui magna cillum ipsum enim aute ex. Sint veniam deserunt id do velit eu.\\r\\n\",\n    \"registered\": \"2016-10-15T11:07:09 -01:00\",\n    \"latitude\": -71.61758,\n    \"longitude\": -73.196318,\n    \"tags\": [\n      \"pariatur\",\n      \"officia\",\n      \"do\",\n      \"est\",\n      \"aute\",\n      \"ipsum\",\n      \"elit\"\n    ],\n    \"friends\": [\n      {\n        \"id\": 0,\n        \"name\": \"Todd Mccray\"\n      },\n      {\n        \"id\": 1,\n        \"name\": \"Carrillo Johns\"\n      },\n      {\n        \"id\": 2,\n        \"name\": \"Claire Evans\"\n      }\n    ],\n    \"greeting\": \"Hello, Pugh Christensen! You have 6 unread messages.\",\n    \"favoriteFruit\": \"strawberry\"\n  },\n  {\n    \"_id\": \"59b53bcb07c3d92599f358a7\",\n    \"index\": 99,\n    \"guid\": \"00eb41e9-cb16-49c9-84da-e139407a70e3\",\n    \"isActive\": true,\n    \"balance\": \"$3,233.68\",\n    \"picture\": \"http://placehold.it/32x32\",\n    \"age\": 37,\n    \"eyeColor\": \"blue\",\n    \"name\": \"Knapp Mccullough\",\n    \"gender\": \"male\",\n    \"company\": \"EARWAX\",\n    \"email\": \"knappmccullough@earwax.com\",\n    \"phone\": \"+1 (987) 583-3507\",\n    \"address\": \"180 Adelphi Street, Grahamtown, New York, 2149\",\n    \"about\": \"Aliquip aliquip enim ullamco minim consectetur consequat qui anim nulla do elit dolor dolore. Mollit mollit cillum aliquip culpa veniam esse dolor commodo aliqua laborum dolor duis culpa. Commodo ex id excepteur ipsum. Aliqua occaecat sunt ipsum aliqua exercitation irure. Nisi commodo eu consequat sit elit occaecat excepteur. Fugiat in ipsum excepteur magna minim eiusmod in eu consectetur minim qui exercitation. Laborum irure est ullamco aliqua consectetur aliqua.\\r\\n\",\n    \"registered\": \"2015-12-19T05:55:46 -00:00\",\n    \"latitude\": 46.042325,\n    \"longitude\": 3.527828,\n    \"tags\": [\n      \"occaecat\",\n      \"exercitation\",\n      \"enim\",\n      \"aliqua\",\n      \"ut\",\n      \"eu\",\n      \"amet\"\n    ],\n    \"friends\": [\n      {\n        \"id\": 0,\n        \"name\": \"Maryanne Finley\"\n      },\n      {\n        \"id\": 1,\n        \"name\": \"Goff Joyce\"\n      },\n      {\n        \"id\": 2,\n        \"name\": \"Scott Callahan\"\n      }\n    ],\n    \"greeting\": \"Hello, Knapp Mccullough! You have 4 unread messages.\",\n    \"favoriteFruit\": \"banana\"\n  }\n]"
  out "Table Control":string[][](table)
  in  "$Path examples (Please select)":string(combo)="$[*].friends[*].name"
  # "Example JSON from https://www.json-generator.com"
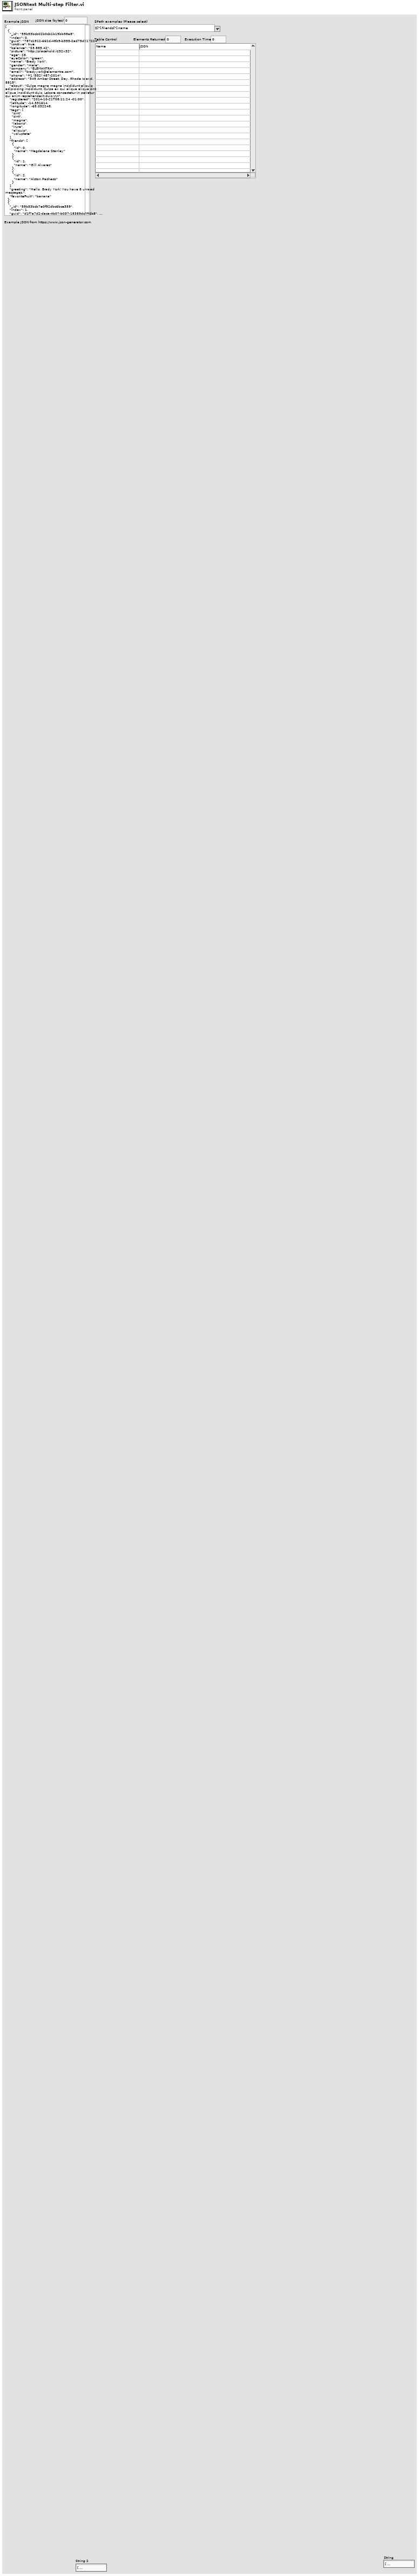
[diagram p1: front panel]
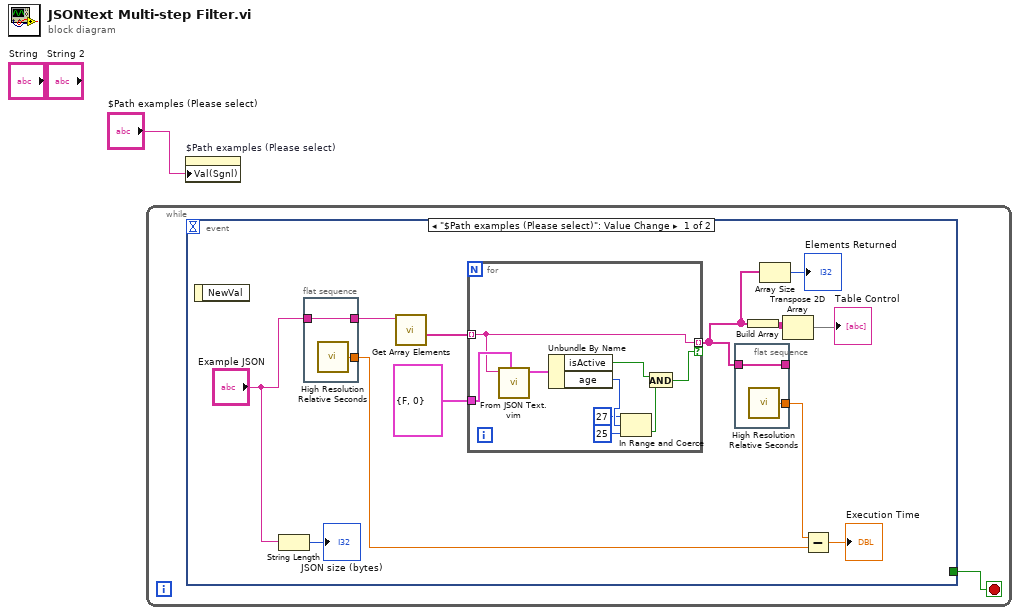
[diagram p0: block diagram]
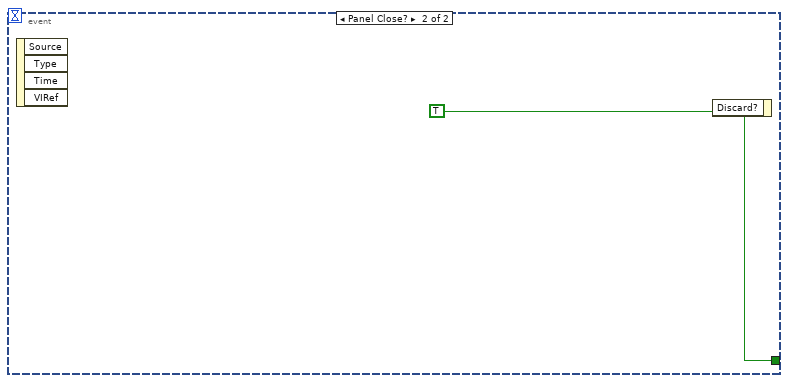
[diagram p2: hidden frame]
diagram:
  n1 = while {
    stop <- w2 stop-if-true
    n2 = event shown="[0] \"$Path examples (Please select)\": Value Change" {
      selector: _ -> [_ _]
      dyn-events: _ -> [_ _]
      timeout: _ -> [_ _]
      tunnel: [_ w28] -> w2
      event "$Path examples (Please select)": Value Change {
        n3 = event-data() -> ()  [unwired: 1 in, 1 out]
        n4 = String Length(string="Example JSON") -> (length=→"JSON size (bytes)":i32)
        n5 = flat-sequence {
          tunnel: "Example JSON" -> [w27]
          tunnel: [w27] -> w6
          tunnel: [w26] -> w11
          frame #0 {
            n6 = call <vilib>:"High Resolution Relative Seconds.vi"() -> ("relative seconds"=w26:dbl)
          }
        }
        n7 = call "Get Array Elements.vi"("JSON"=w6) -> ("<JSON>"=w5:string[])  [unwired: 8 in, 2 out]
        n8 = for {
          tunnel: [w16] -> w3 mode=indexing if=w15
          tunnel: w5 -> [w16] mode=indexing
          tunnel: cluster{"isActive":bool, "age":i32} {"isActive"=FALSE, "age"=0} -> [w23]
          n9 = call "From JSON Text.vim"("Data Type and Default Value"=w23, "JSON"=w16) -> ("Variant out"=w22:cluster{"isActive":bool, "age":i32})  [unwired: 8 in, 1 out]
          n10 = Unbundle By Name(w22) -> ("isActive"=w21:bool, "age"=w20:i32)
          n11 = In Range and Coerce(upper limit=27, x=w20, lower limit=25) -> (In Range?=w17:bool)  [unwired: 1 out]
          n12 = And(x=w21, y=w17) -> (x .and. y?=w15:bool)
        }
        n13 = flat-sequence {
          tunnel: w3 -> [w25]
          tunnel: [w25] -> _
          tunnel: [w24] -> w12
          frame #0 {
            n14 = call <vilib>:"High Resolution Relative Seconds.vi"() -> ("relative seconds"=w24:dbl)
          }
        }
        n15 = Build Array(w3) -> (w14:string[][])
        n16 = Array Size(array=w3) -> (size(s)=→"Elements Returned":i32)
        n17 = Transpose 2D Array(2D array=w14) -> (transposed array=→"Table Control":string[][])
        n18 = Subtract(x=w12, y=w11) -> (x-y=→"Execution Time":dbl)
      }
      event Panel Close? {
        w28 = TRUE
        n19 = event-data() -> ()  [unwired: 1 in, 4 out]
        n20 = event-data("Discard?"=w28) -> ()  [unwired: 1 in, 1 out]
      }
    }
  }
  n21 = property on="$Path examples (Please select)" class="CmbBox"("Val(Sgnl)"="$Path examples (Please select)") -> ()  [unwired: 2 in, 2 out]
